vi "EDGE-TRIGGERED-D-TYPE-FLIP-FLOP.vi"(2 "WRITE":bool) -> (0 "Q-bar":bool)   [LabVIEW 2014]
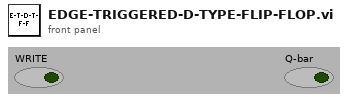
[diagram p1: front panel]
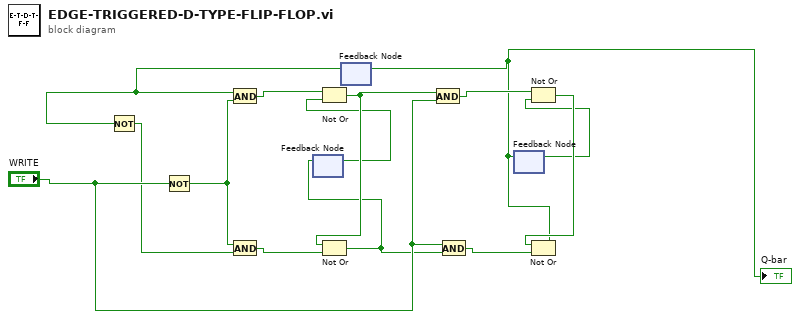
[diagram p0: block diagram]
diagram:
  n1 = Not(x="WRITE") -> (.not. x?=w9:bool)
  n2 = feedback #1() -> (w5:bool)  [unwired: 1 out]
  n3 = feedback #2() -> (w2:bool)  [unwired: 1 in]
  n4 = Not(x=w2) -> (.not. x?=w6:bool)
  n5 = And(x=w2, y=w9) -> (x .and. y?=w3:bool)
  n6 = And(x=w9, y=w6) -> (x .and. y?=w4:bool)
  n7 = Not Or(1:w5, 2:w3) -> (0:w8:bool)
  n8 = Not Or(1:w4, 2:w8) -> (0:w7:bool)
  n9 = feedback-in #1(w7) -> ()
  n10 = And(x=w8, y="WRITE") -> (x .and. y?=w11:bool)
  n11 = And(x="WRITE", y=w7) -> (x .and. y?=w12:bool)
  n12 = feedback #3() -> (w13:bool)  [unwired: 1 out]
  n13 = Not Or(1:w13, 2:w11) -> (0:w14:bool)
  n14 = Not Or(1:w12, 2:w14) -> (0:w1:bool)
  "Q-bar" <- w1
  n15 = feedback-in #2(w1) -> ()
  n16 = feedback-in #3(w1) -> ()
